vi "Write State Data to Datalog.vi"(8 "error in (no error)":errorcluster, 11 "Base Step in":refnum<class "Base Step.lvclass">) -> (0 "error out":errorcluster)   [LabVIEW 2024, in "Ramses Sequencer.lvlib" / "Base Step.lvclass"]
uses:
  Base Step.lvclass
  Base Step.lvclass/Base Step.ctl
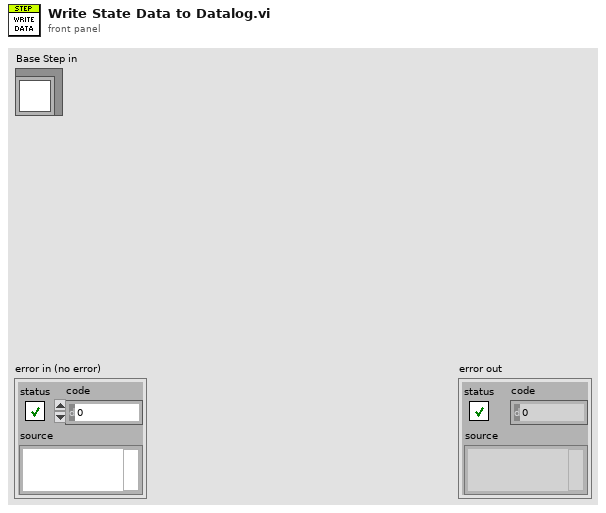
[diagram p1: front panel]
types:
  T1 = typedef "Ramses Sequencer.lvlib/Base Step.lvclass/Step State.ctl" = cluster{"Result":string, "Status":string, "Enabled":bool, "Upper":string, "Target":string, "Lower":string, "Value":string}
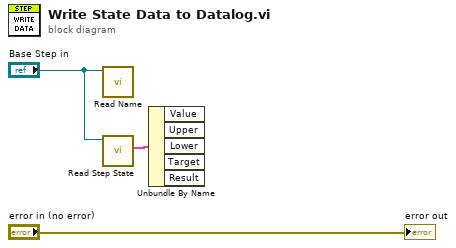
[diagram p0: block diagram]
diagram:
  n1 = call-dynamic "Read Name.vi"("Base Step in"="Base Step in") -> ()  [unwired: 8 in, 3 out]
  n2 = call "Read Step State.vi"("Base Step in"="Base Step in") -> ("Step State"=w3:T1)  [unwired: 8 in, 2 out]
  n3 = Unbundle By Name(w3) -> ()  [unwired: 5 out]
  "error out" <- "error in (no error)"
